vi "Download iconlibrary files.vi"(8 "error in":errorcluster) -> (0 "error out":errorcluster, 2 "Unzipped files":path[](array[path]), 3 "parent path":path, 4 "Cancelled?":bool, 5 "XML Data":T1[](array[typedef]))   [LabVIEW 2020, in "lv_icon.lvlib"]
uses:
  lv_icon.lvlib
  <vilib>/zip/NI_Unzip.lvlib
  Controls/XMLDataStructureIconLibrary.ctl
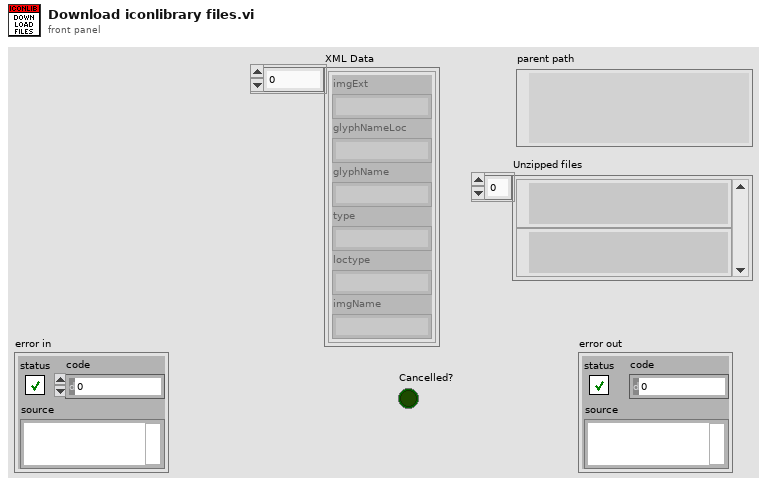
[diagram p1: front panel]
types:
  T1 = typedef "XMLDataStructureIconLibrary.ctl" = cluster{"imgExt":string, "glyphNameLoc":string, "glyphName":string, "type":string, "loctype":string, "imgName":string}
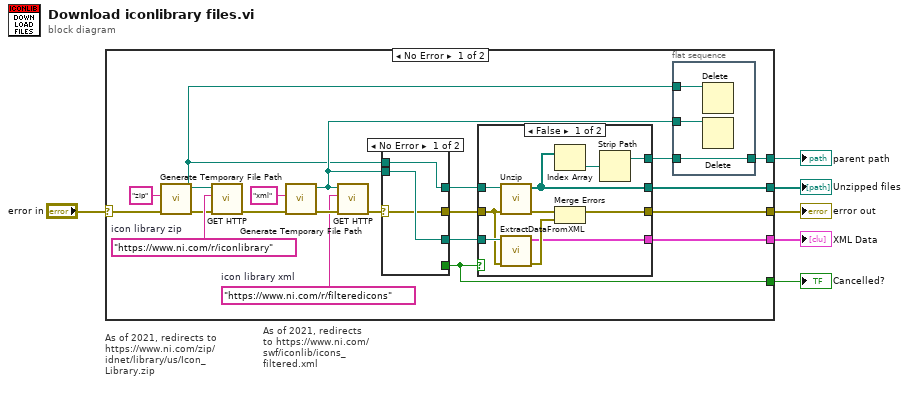
[diagram p0: block diagram]
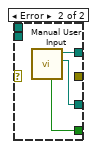
[diagram p3: hidden frame]
diagram:
  # "As of 2021, redirects to https://www.ni.com/swf/iconlib/icons_filtered.xml"
  # "As of 2021, redirects to https://www.ni.com/zip/idnet/library/us/Icon_Library.zip"
  n1 = case shown="No Error" "error in" {
    selector: "error in" -> [w18 w47]
    tunnel: [w26 _] -> w1
    tunnel: [w14 _] -> w5
    tunnel: [w24 _] -> w4
    tunnel: [w23 w47] -> w3
    tunnel: [w16 _] -> w2
    frame No Error {
      w9 = "https://www.ni.com/r/filteredicons"  # icon library xml
      w11 = "https://www.ni.com/r/iconlibrary"  # icon library zip
      n2 = call <vilib>:"Generate Temporary File Path.vi"("error in (no error)"=w18, "Temporary File Extension (tmp)"="zip") -> ("error out"=w8:errorcluster, "Unique Temporary File Path"=w7:path)  [unwired: 8 in]
      n3 = call "GET HTTP.vi"("error in (no error)"=w8, "URL"=w11, "output file"=w7) -> ("error out"=w17:errorcluster)  [unwired: 8 in]
      n4 = call <vilib>:"Generate Temporary File Path.vi"("error in (no error)"=w17, "Temporary File Extension (tmp)"="xml") -> ("error out"=w13:errorcluster, "Unique Temporary File Path"=w10:path)  [unwired: 8 in]
      n5 = call "GET HTTP.vi"("error in (no error)"=w13, "URL"=w9, "output file"=w10) -> ("error out"=w12:errorcluster)  [unwired: 8 in]
      n6 = case shown="No Error" w12 {
        selector: w12 -> [w41 _]
        tunnel: w7 -> [w43 _]
        tunnel: [w43 w45] -> w25
        tunnel: w10 -> [w42 _]
        tunnel: [_ w46] -> w26
        tunnel: [w41 _] -> w22
        tunnel: [w42 w44] -> w21
        frame No Error {
        }
        frame Error {
          n7 = call "Manual User Input.vi"() -> ("XML"=w44:path, "ZIP"=w45:path, "Cancelled?"=w46:bool)  [unwired: 9 in]
        }
      }
      n8 = case shown="False" w26 {
        tunnel: w25 -> [w38 _]
        tunnel: [w37 _] -> w15
        tunnel: [w36 _] -> w24
        tunnel: [w34 w40] -> w23
        tunnel: w22 -> [w30 w40]
        tunnel: w21 -> [w33 _]
        tunnel: [w31 _] -> w16
        frame False {
          n9 = call <vilib>:"Unzip.vi"("error in (no error)"=w30, "Zip file"=w38) -> ("error out"=w35:errorcluster, "Unzipped files"=w36:path[])  [unwired: 2 in, 6 out]
          n10 = call "ExtractDataFromXML.vi"("error in (no error)"=w30, "path to XML document"=w33) -> ("error out"=w32:errorcluster, "XML Data"=w31:T1[])  [unwired: 8 in]
          n11 = Index Array(array=w36) -> (element=w39:path)  [unwired: 1 in]
          n12 = Merge Errors(w35, w32) -> (w34:errorcluster)
          n13 = Strip Path(path=w39) -> (stripped path=w37:path)  [unwired: 1 out]
        }
        frame True {
        }
      }
      n14 = flat-sequence {
        tunnel: w7 -> [w29]
        tunnel: w15 -> [w28]
        tunnel: [w28] -> w14
        tunnel: w10 -> [w27]
        frame #0 {
          n15 = Delete(path (use dialog)=w29) -> ()  [unwired: 4 in, 3 out]
          n16 = Delete(path (use dialog)=w27) -> ()  [unwired: 4 in, 3 out]
        }
      }
    }
    frame Error {
    }
  }
  "Unzipped files" <- w4
  "error out" <- w3
  "parent path" <- w5
  "Cancelled?" <- w1
  "XML Data" <- w2
